vi "testUIPanelOpenifpreviouslyOpen.vi"(8 "error in (no error)":errorcluster, 11 "testStateMachineUtilities in":refnum<class "testStateMachineUtilities.lvclass">) -> (0 "error out":errorcluster, 3 "testStateMachineUtilities out":refnum<class "testStateMachineUtilities.lvclass">)   [LabVIEW 2013, in "testStateMachineUtilities.lvclass"]
uses:
  testStateMachineUtilities.lvclass
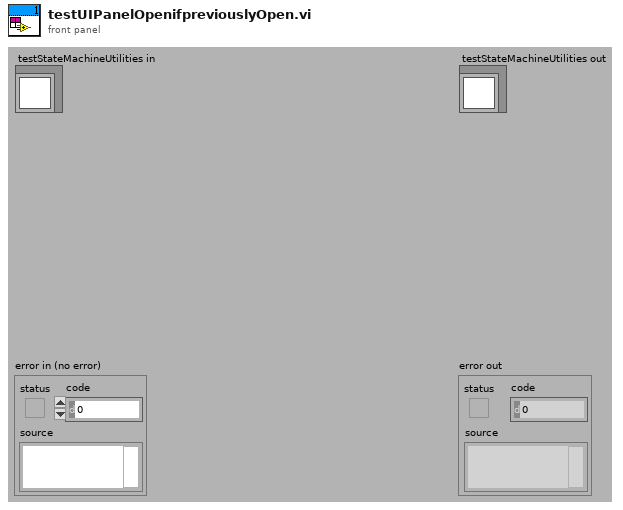
[diagram p1: front panel]
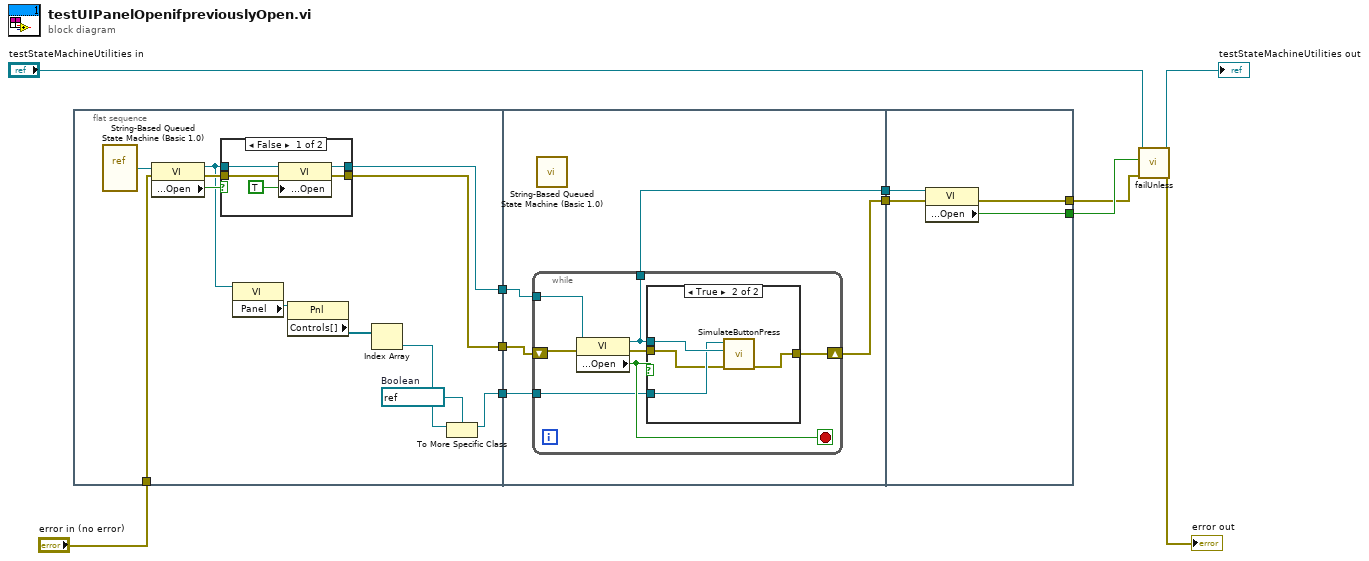
[diagram p0: block diagram]
diagram:
  n1 = flat-sequence {
    tunnel: [w20] -> w8
    tunnel: [w19] -> w3
    tunnel: "error in (no error)" -> [w18]
    tunnel: [w12] -> w1
    tunnel: w8 -> [w35]
    tunnel: [w34] -> w7
    tunnel: [w33] -> w4
    tunnel: w3 -> [w32]
    tunnel: w1 -> [w31]
    tunnel: w7 -> [w51]
    tunnel: [w48] -> w6
    tunnel: [w50] -> w5
    tunnel: w4 -> [w49]
    frame #0 {
      w13 = refnum<vi> refnum  # Boolean
      n2 = vi-ref "String-Based Queued State Machine (Basic 1.0).vi"() -> (w21:refnum<vi>)
      n3 = property class="VI"(reference=w21, error in=w18) -> (reference out=w17:refnum<vi>, error out=w23:errorcluster, "Front Panel.Open"=w22:bool)
      n4 = case shown="False" w22 {
        tunnel: w17 -> [w28 w30]
        tunnel: w23 -> [w26 w29]
        tunnel: [w25 w30] -> w20
        tunnel: [w24 w29] -> w19
        frame False {
          n5 = property class="VI"(reference=w28, error in=w26, "Front Panel.Open"=TRUE ("Front Panel Window:Open")) -> (reference out=w25:refnum<vi>, error out=w24:errorcluster)
        }
        frame True {
        }
      }
      n6 = property class="VI"(reference=w17) -> ("Panel"=w16:refnum<vi>)  [unwired: 1 in, 2 out]
      n7 = property class="Pnl"(reference=w16) -> ("Controls[]"=w15:refnum<vi>[])  [unwired: 1 in, 2 out]
      n8 = Index Array(array=w15) -> (element=w14:refnum<vi>)  [unwired: 1 in]
      n9 = To More Specific Class(target class=w13, reference=w14) -> (specific class reference=w12:refnum<vi>)  [unwired: 1 in, 1 out]
    }
    frame #1 {
      n10 = while {
        tunnel: w35 -> [w42]
        tunnel: [w37] -> w34
        shift-right: [w40] -> w33
        shift-left: w32 -> [w39]
        tunnel: w31 -> [w36]
        stop <- w41 stop-if-true
        n11 = property class="VI"(reference=w42, error in=w39) -> (reference out=w37:refnum<vi>, error out=w38:errorcluster, "Front Panel.Open"=w41:bool)
        n12 = case shown="True" w41 {
          tunnel: [w43 w45] -> w40
          tunnel: w38 -> [w43 w44]
          tunnel: w37 -> [_ w47]
          tunnel: w36 -> [_ w46]
          frame False {
          }
          frame True {
            n13 = call "SimulateButtonPress.vi"("error in (no error)"=w44, "VIRef"=w47, "BooleanCtrlRef"=w46) -> ("error out"=w45:errorcluster)  [unwired: 8 in]
          }
        }
      }
      n14 = call "String-Based Queued State Machine (Basic 1.0).vi"() -> ()  [unwired: 1 in]
    }
    frame #2 {
      n15 = property class="VI"(reference=w51, error in=w49) -> (error out=w50:errorcluster, "Front Panel.Open"=w48:bool)  [unwired: 1 out]
    }
  }
  n16 = call-dynamic "failUnless.vi"("error in (no error)"=w5, "pass"=w6, "TestCase in"="testStateMachineUtilities in") -> ("error out"=→"error out":errorcluster, "TestCase out"=→"testStateMachineUtilities out":refnum<class "testStateMachineUtilities.lvclass">)  [unwired: 7 in]
